vi "calibrationElectrometer_logEvent_largeFileObjectAvailable.vi"(8 "error in (no error)":errorcluster, 11 "logevent_largeFileObjectAvailable_Ctl":T1={"url"="", "generator"="", "version"=0.0, "checkSum"="", "mimeType"="                                ", "byteSize"=0, "id"="", "priority"=0}) -> (0 "error out":errorcluster, 2 "function return":i32, 3 "logevent_largeFileObjectAvailable_Ctl out":T1={"url"="", "generator"="", "version"=0.0, "checkSum"="", "mimeType"="                                ", "byteSize"=0, "id"="", "priority"=0})   [LabVIEW 2016, in "SALLV_calibrationElectrometer.lvlib"]
doc: "int calibrationElectrometer_shm_logEvent_largeFileObjectAvailableLV(calibrationElectrometer_logevent_largeFileObjectAvailableLV *logevent_largeFileObjectAvailable_Ctl );"
uses:
  SALLV_calibrationElectrometer.lvlib
  DataTypes/logevent_largeFileObjectAvailable.ctl
  SALLV_calibrationElectrometer.so
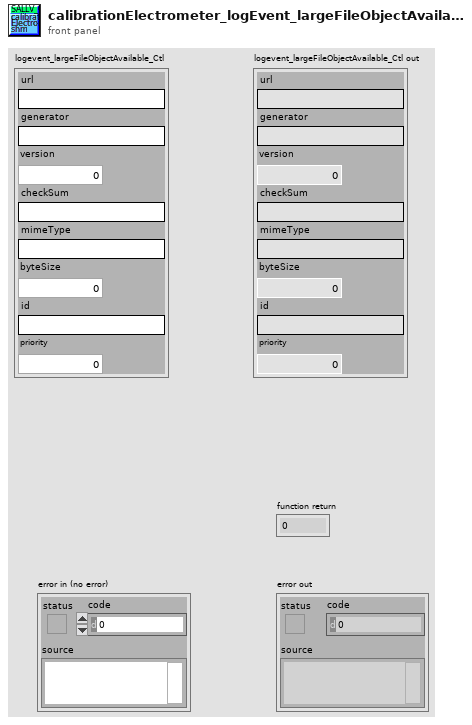
[diagram p1: front panel]
types:
  T1 = typedef "SALLV_calibrationElectrometer.lvlib/logevent_largeFileObjectAvailable.ctl" = cluster{"url":string, "generator":string, "version":sgl, "checkSum":string, "mimeType":string, "byteSize":i32, "id":string, "priority":i32}
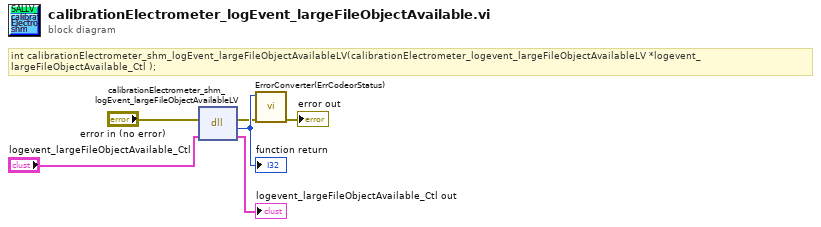
[diagram p0: block diagram]
diagram:
  # "int calibrationElectrometer_shm_logEvent_largeFileObjectAvailableLV(calibrationElectrometer_logevent_largeFileObjectAvailableLV *logevent_largeFileObjectAvailable_Ctl );"
  n1 = dll-call lib="home/andres/Desktop/SAL_calibrationElectrometer/SALLV_calibrationElectrometer.*" fn="calibrationElectrometer_shm_logEvent_largeFileObjectAvailableLV"(error in="error in (no error)", "logevent_largeFileObjectAvailable_Ctl"="logevent_largeFileObjectAvailable_Ctl") -> (error out=w2:errorcluster, w6:i32, "logevent_largeFileObjectAvailable_Ctl"=→"logevent_largeFileObjectAvailable_Ctl out":T1)  [unwired: 2 in, 1 out]
  "function return" <- w6
  n2 = call "ErrorConverter(ErrCodeorStatus).vi"("error in (no error)"=w2, "error code"=w6) -> ("error out"=→"error out":errorcluster)  [unwired: 9 in]
